vi "APVSG20 module.vi"(10 "Supramodle mailbox":T3) -> ()   [LabVIEW 2024, in "THz source modeule.lvlib"]
doc: "This is a 2024 gen. module for control of AnaPico vector signal generator. \n\nObsolate notes:\nKey typedefs: THz_Message for module, THz_Comands enum (Ignore, Initialize, Update, Set parameters, Disconnect, End), THz_Sweeep parameters\n\nComands and responses:\nInitialize: VDI config constants {Master{lower limit, upper limit, name, handle, description}, Follower{ lower limit, upper limit, name, handle, description } } (cluster of two clusters {numeric, numeric, string, numeric, string}) / handle log (string)\nUpdate: - / M_ID F_ID (string)\nSet parameters: Sweep parameters {Start, End, Sweep up time, Sweep down time, Intermediate, Reset trigger} (cluster{numeric, numeric, numeric, numeric, numeric, boolean}) / Sweep parameters (same cluster)\nDisconnect: - / master and follower name (string)\nEnd: - / Master and Follower handle (string)"
uses:
  THz source modeule.lvlib
  Messenger service/Data types/Module name.ctl
  <vilib>/ErrorRing/Error Ring.xnode
  ctl/APVSG module action.ctl
  <userlib>/MatS Libs/MatS Libs.lvlib
  <userlib>/MatS Libs/MatS Mailman/TypeDefs/General message.ctl
  Magnet module/ctl/Tmp_M commands.ctl
  Magnet module/Magnet module.lvlib
  <userlib>/MatS Libs/MatS Mailman/TypeDefs/Mailbox ref.ctl
  ctl/THz MW generator constants.ctl
  ctl/Module status.ctl
  ctl/THz commands enum.ctl
  <instrlib>/APVSG/APVSG20.lvlib
panel:
  out "Instrument status":T1={"Lower limit [GHz]"=8.0, "Upper limit [GHz]"=20.0, "Device name"="VDIYT7", "Connection"="", "Description"="VDI Tracking", "Connected"=FALSE, "Last settings"="", "Operation mode"=enum."Disabled", "Enable ch 1"=FALSE, "Enable ch 2"=FALSE}
  out "Modul status":T2={"Supramodule"=refnum, "This module"=refnum, "Submodule"=refnum, "Module name"="", "Is standalone"=FALSE, "Timer [ms]"=0, "Reset timer"=TRUE, "Last change"=timestamp(0 s since 1904-01-01), "Logs"=[], "Ended"=FALSE} {"Last change" format="%<%H:%M:%S\n%Y/%m/%d>T"}
  in  "This module mailbox":refnum<queue>
  in  "APVSG tab":enum32{"Status", "CW", "Sweep", "Arbitrary"}(tab)
  in  "Exit APVSG btn":bool
  in  "Connect btn":bool
  in  "Enable ch 2":bool
  in  "Enable ch 1":bool
  in  "VISA resource name":refnum<visa-resource-name>
  out "Is connected":bool
  in  "CW settings":T4(array[cluster])
  in  "Sweep table":T5(array[cluster])
  in  "Waveform files":path[](array[path])
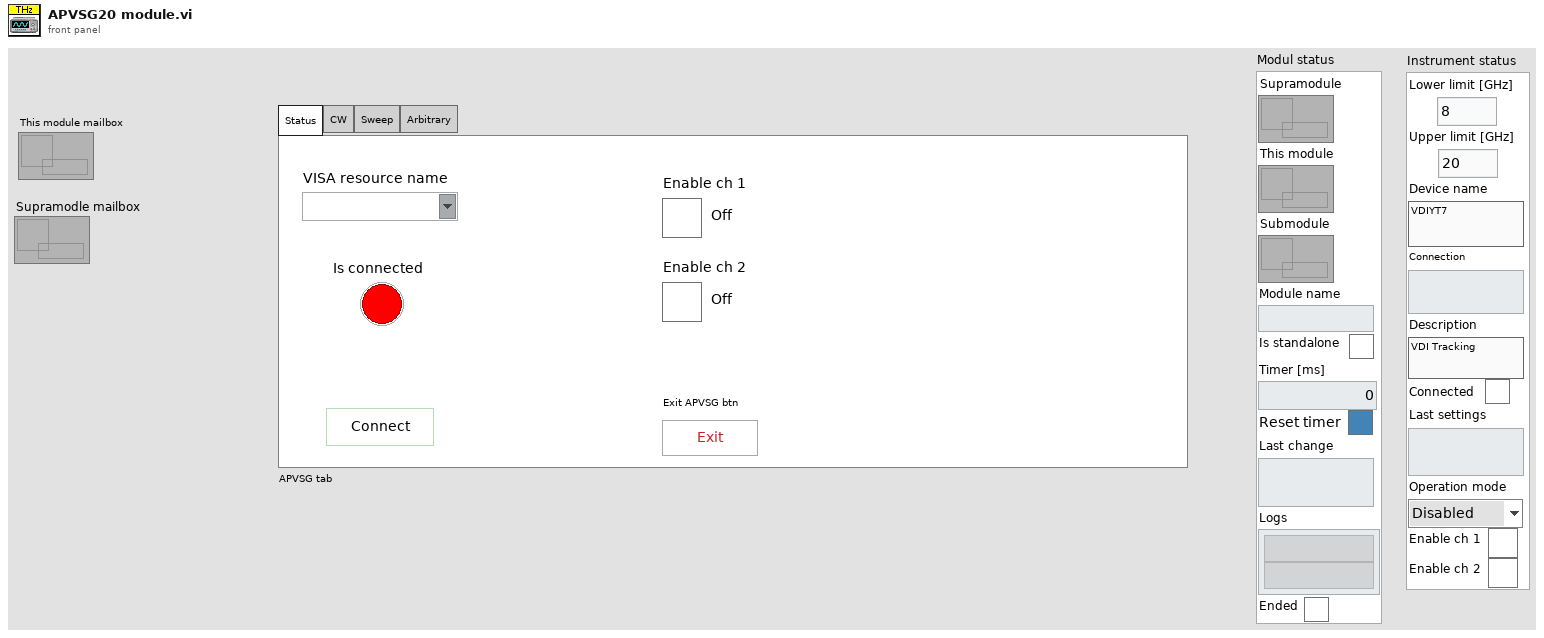
[diagram p1: front panel]
types:
  T1 = typedef "THz source modeule.lvlib/THz MW generator constants.ctl" = cluster{"Lower limit [GHz]":dbl, "Upper limit [GHz]":dbl, "Device name":string, "Connection":string, "Description":string, "Connected":bool, "Last settings":string, "Operation mode":enum16{"Disabled", "CW", "Arbitrary", "Sweep"}, "Enable ch 1":bool, "Enable ch 2":bool}
  T2 = typedef "THz source modeule.lvlib/Module status.ctl" = cluster{"Supramodule":T3, "This module":T3, "Submodule":T3, "Module name":string, "Is standalone":bool, "Timer [ms]":i32, "Reset timer":bool, "Last change":timestamp, "Logs":string[], "Ended":bool}
  T3 = typedef "MatS Libs.lvlib/Mailbox ref.ctl" = refnum<queue>
  T4 = cluster{"Frequency (GHz)":dbl, "Amplitude (dBm)":dbl}[]
  T5 = cluster{"Frequency (GHz)":dbl, "Amplitude (dBm)":dbl, "Time (ns)":dbl}[][]
  T6 = typedef "Module name.ctl" = enum16{"Emty", "Magnet", "VTI", "Excitation", "Servo", "Acquisition", "Rotator", "Digitizer", "SMU2450", "Carousel", "Multimeter", "Tmp monitor", "Power monitor"}
  T7 = cluster{"Supramodule":T3, "This module":T3, "Module name":string, "Standalone?":bool, "Stopped?":bool, "Instr reference":string, "Connected?":bool, "Last update":timestamp, "Logs":string[], "Update period ms":u32}
  T8 = enum16{"Initialize", "Wait for event", "Check message", "Check changes", "End"}
  T9 = typedef "THz source modeule.lvlib/APVSG module action.ctl" = enum16{"Initialize", "Check cmd", "Wait for event", "Connect", "Disconnect", "Query instr", "Set CW", "Set sweep", "Set waveform", "Enable output", "Disable output", "Exit"}
  T10 = enum32{"Bad", "Idle", "Run top level", "Running"}
  T11 = typedef "Magnet module.lvlib/Tmp_M commands.ctl" = enum16{"Ignore", "Log", "Connect", "Set timeout", "Update", "Disconnect", "End"}
  T12 = typedef "MatS Libs.lvlib/General message.ctl" = cluster{"Sender":string, "Recipient":string, "Topic":variant, "Content":variant, "Time Stamp":timestamp}
  T13 = enum16{"Ignore", "Log", "Connect", "Set timeout", "Update", "Disconnect", "End"}
  T14 = enum16{"Ignore", "Log", "Connect", "Set timeout", "Update", "Disconnect", "End"}[]
  T15 = typedef "THz source modeule.lvlib/THz commands enum.ctl" = enum16{"Ignore", "Connect", "Update", "Set parameters", "Disconnect", "End"}
  T16 = enum8{"Enabled", "Disabled", "Disabled and Grayed Out"}
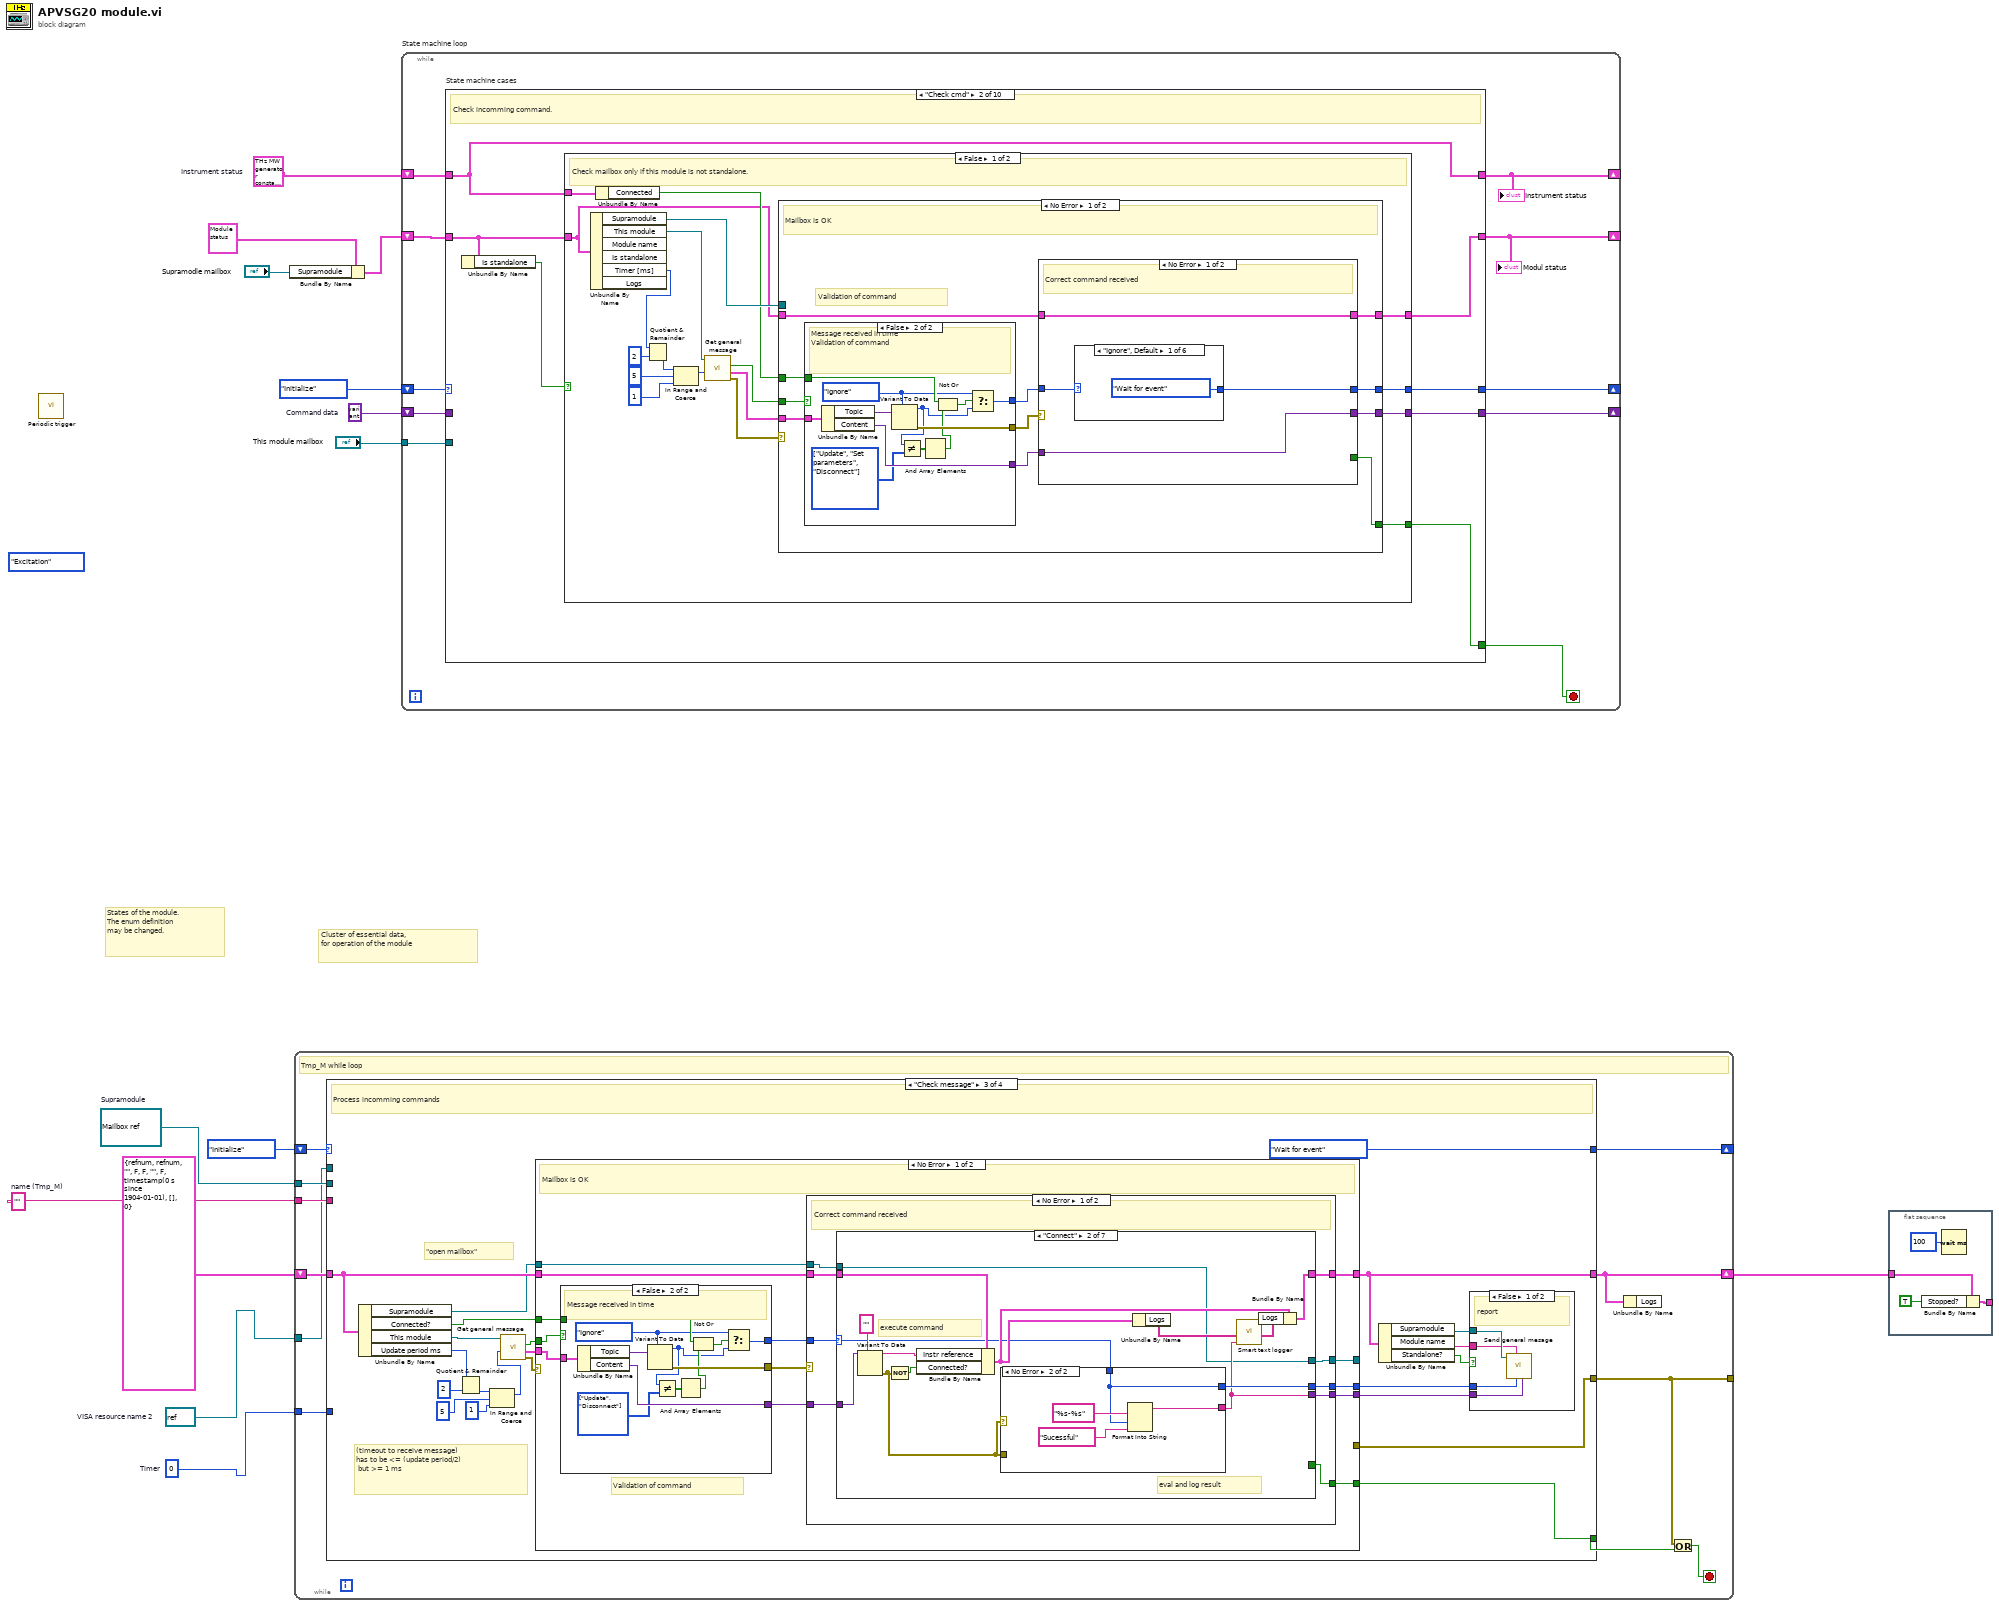
[diagram p0: block diagram]
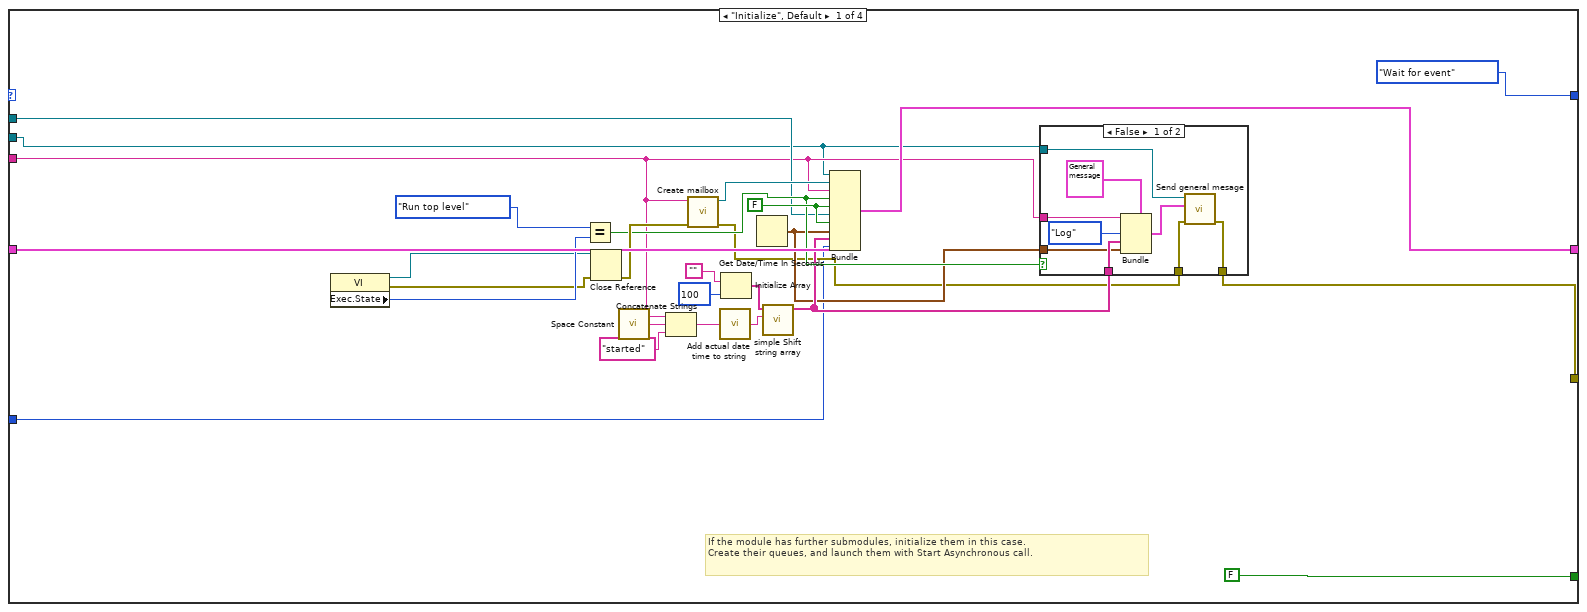
[diagram p2: hidden frame]
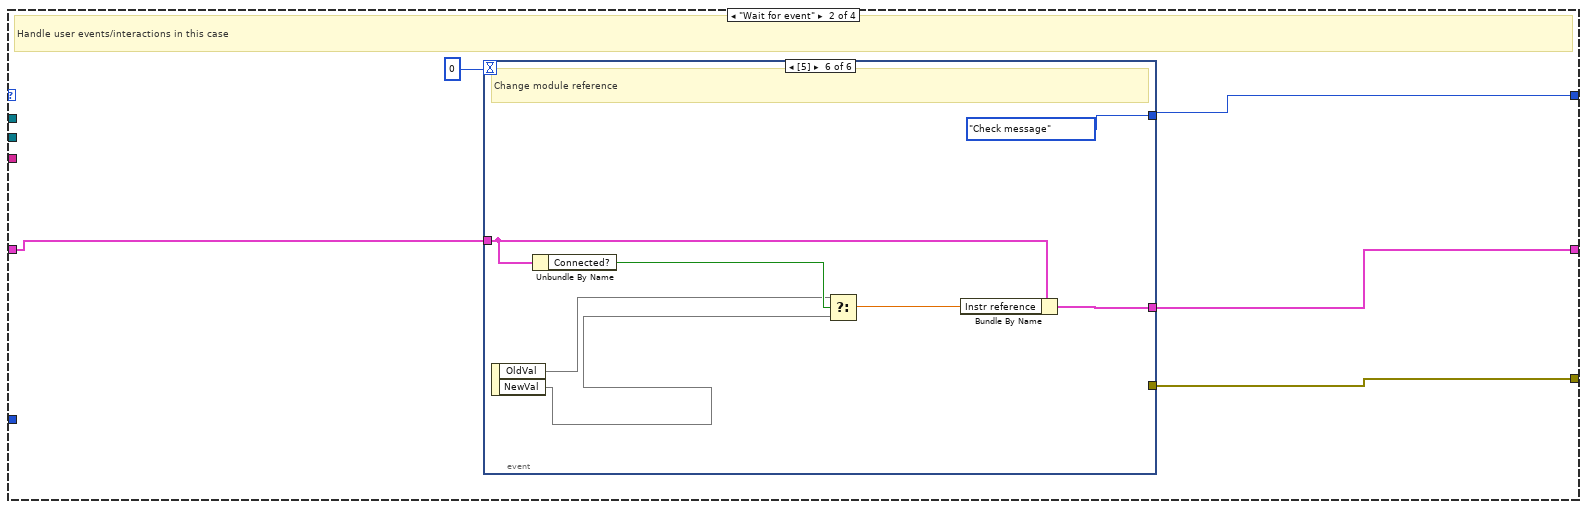
[diagram p4: hidden frame]
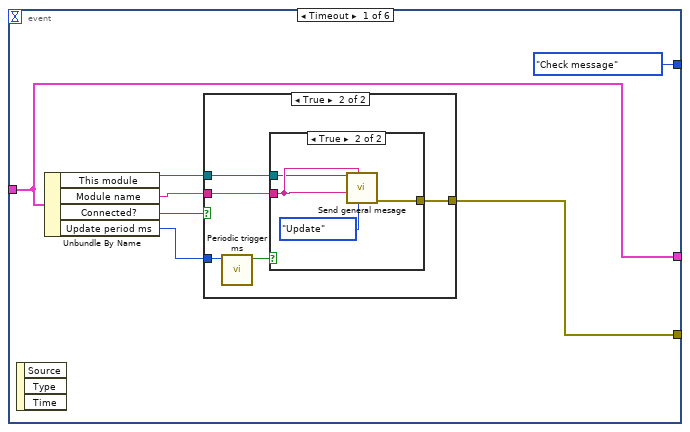
[diagram p5: hidden frame]
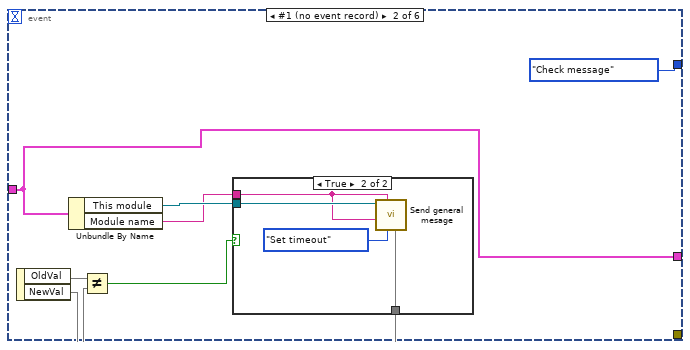
[diagram p8: hidden frame]
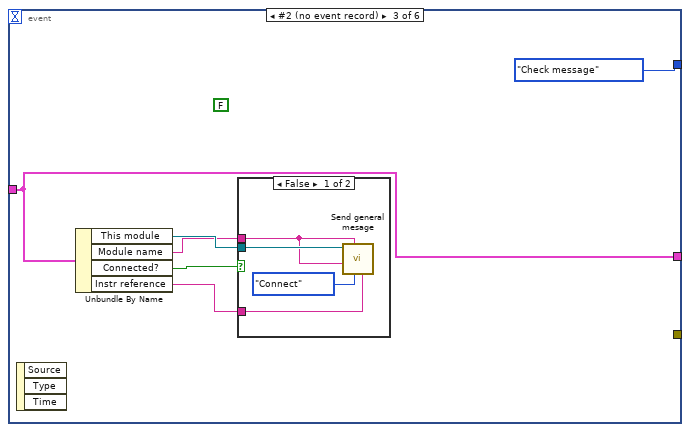
[diagram p10: hidden frame]
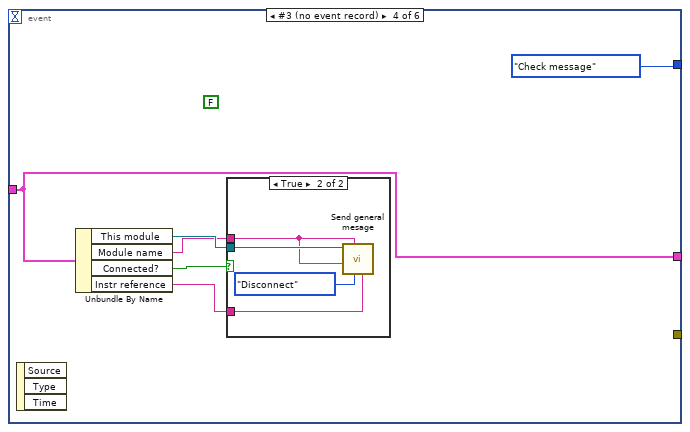
[diagram p12: hidden frame]
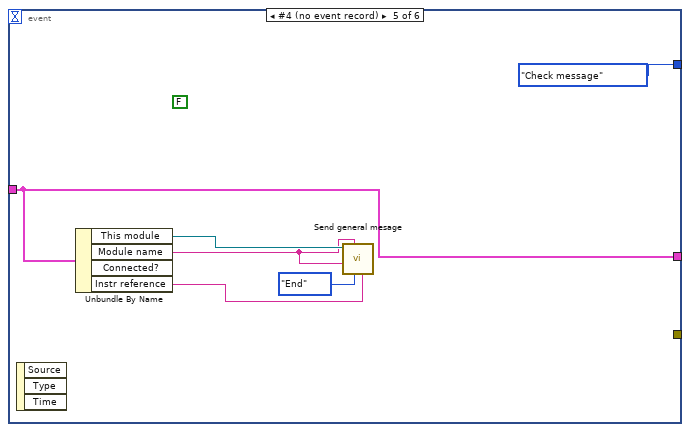
[diagram p14: hidden frame]
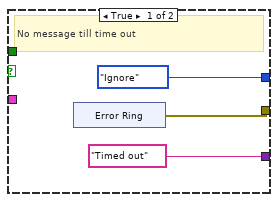
[diagram p16: hidden frame]
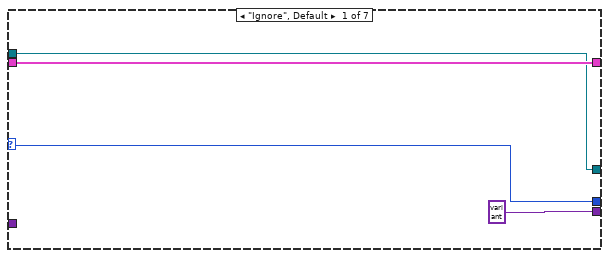
[diagram p17: hidden frame]
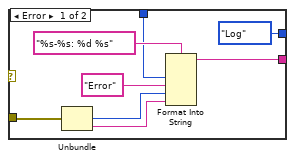
[diagram p18: hidden frame]
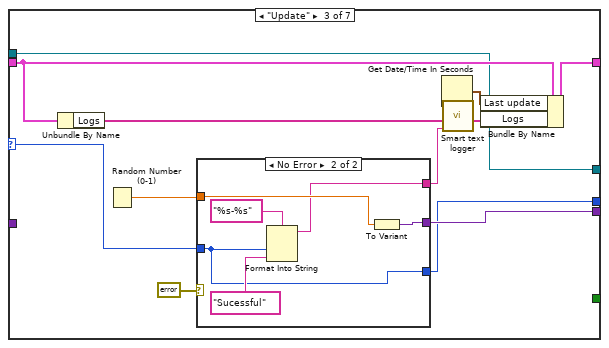
[diagram p19: hidden frame]
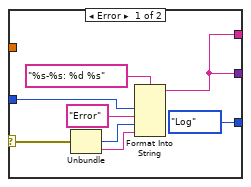
[diagram p20: hidden frame]
diagram:
  (unwired) Module_name."Excitation" ("Module")
  w3 = T1 {"Lower limit [GHz]"=8.0, "Upper limit [GHz]"=20.0, "Device name"="VDIYT7", "Connection"="", "Description"="VDI Tracking", "Connected"=FALSE, "Last settings"="", "Operation mode"=enum."Disabled", "Enable ch 1"=FALSE, "Enable ch 2"=FALSE}  # Instrument status
  w4 = variant  # Command data
  w11 = 0  # Timer
  w10 = refnum<visa-resource-name> refnum  # VISA resource name 2
  w9 = ""  # name (Tmp_M)
  w8 = T3 refnum  # Supramodule
  # "States of the module.\nThe enum definition\nmay be changed."
  # "Cluster of essential data,\nfor operation of the module"
  n1 = call <userlib>:"Periodic trigger.vi"() -> ()  [unwired: 3 in, 1 out]
  n2 = Bundle By Name(cluster=T2 {"Supramodule"=refnum, "This module"=refnum, "Submodule"=refnum, "Module name"="Signal generator", "Is standalone"=FALSE, "Timer [ms]"=5000, "Reset timer"=FALSE, "Last change"=timestamp(0 s since 1904-01-01), "Logs"=[], "Ended"=FALSE}, "Supramodule"="Supramodle mailbox") -> (w2:T2)
  n3 = while {
    tunnel: [w19] -> _
    shift-right: [w23] -> _
    shift-left: T8."Initialize" -> [w24]
    shift-right: [w20] -> w6
    shift-left: T7 {"Supramodule"=refnum, "This module"=refnum, "Module name"="", "Standalone?"=FALSE, "Stopped?"=FALSE, "Instr reference"="", "Connected?"=FALSE, "Last update"=timestamp(0 s since 1904-01-01), "Logs"=[], "Update period ms"=0} ("Module status") -> [w22]
    tunnel: w9 -> [w18]
    tunnel: w8 -> [w17]
    tunnel: w11 -> [w16]
    tunnel: w10 -> [w15]
    stop <- w21 stop-if-true
    # "Tmp_M while loop"
    n4 = case shown="\"Check message\"" w24 {
      tunnel: [FALSE _ w149 _] -> w25
      tunnel: [w30 w65 w130 _] -> w19
      tunnel: [T8."Wait for event" w67 T8."Wait for event" T8."End"] -> w23
      tunnel: w22 -> [w50 w63 w147 w374]
      tunnel: [w48 w64 w133 w374] -> w20
      tunnel: w15 -> [w29 _ _ _]
      tunnel: w18 -> [w28 _ _ _]
      tunnel: w17 -> [w27 _ _ _]
      tunnel: w16 -> [w26 _ _ _]
      frame "Initialize", Default {
        w47 = FALSE ("Connected?")
        # "If the module has further submodules, initialize them in this case.\nCreate their queues, and launch them with Start Asynchronous call."
        n5 = property class="VI"() -> (reference out=w38:refnum<vi>, error out=w37:errorcluster, "Exec.State"=w40:T10)  [unwired: 2 in]
        n6 = Equal?(x=T10."Run top level" ("y"), y=w40) -> (x = y?=w34:bool)
        n7 = Close Reference(reference=w38, error in (no error)=w37) -> (error out=w36:errorcluster)
        n8 = call <vilib>:"Space Constant.vi"() -> ("String"=w46:string)
        n9 = Concatenate Strings(w28, w46, "started") -> (w45:string)
        n10 = call <userlib>:"Create mailbox.vi"("error in (no error)"=w36, "name (unnamed)"=w28) -> ("error out"=w31:errorcluster, "Mailbox ref"=w49:T3)  [unwired: 3 in, 1 out]
        n11 = call <userlib>:"Add actual date time to string.vi"("String in"=w45) -> ("String out"=w35:string)  [unwired: 4 in]
        n12 = Initialize Array("", 100 ("dimension size")) -> (w41:string[])
        n13 = Get Date/Time In Seconds() -> (seconds since 1Jan1904=w32:timestamp)
        n14 = call <userlib>:"simple Shift string array.vi"("Element in"=w35, "Array in"=w41) -> ("Array out"=w33:string[])  [unwired: 8 in, 1 out]
        n15 = Bundle(cluster=w50, "Supramodule"=w27, "This module"=w49, "Module name"=w28, "Standalone?"=w34, "Stopped?"=w47, "Instr reference"=w29, "Connected?"=w47, "Last update"=w32, "Logs"=w33, "Update period ms"=w26) -> (w48:T7)
        n16 = case shown="False" w34 {
          tunnel: w27 -> [w61 _]
          tunnel: w33 -> [w59 _]
          tunnel: w32 -> [w58 _]
          tunnel: w28 -> [w56 _]
          tunnel: w31 -> [w55 w62]
          tunnel: [w54 w62] -> w30
          frame False {
            n17 = Bundle(cluster=T12 {"Sender"="", "Recipient"="", "Topic"=variant(string ""), "Content"=variant, "Time Stamp"=timestamp(0 s since 1904-01-01)} ("Message"), "Sender"=w56, "Topic"=Tmp_M_commands."Log" ("Command"), "Content"=w59, "Time Stamp"=w58) -> (w57:T12)  [unwired: 1 in]
            n18 = call <userlib>:"Send general mesage.vi"("error in (no error)"=w55, "Message"=w57, "Mailbox ref in"=w61) -> ("error out"=w54:errorcluster)  [unwired: 6 in, 2 out]
          }
          frame True {
          }
        }
      }
      frame "Wait for event" {
        # "Handle user events/interactions in this case"
        n19 = event shown="[5]" {
          selector: _ -> [_ _ _ _ _ _]
          dyn-events: _ -> [_ _ _ _ _ _]
          timeout: 0 -> [_ _ _ _ _ _]
          tunnel: [T8."Check message" T8."Check message" T8."Check message" T8."Check message" T8."Check message" T8."Check message"] -> w67
          tunnel: [w73 _ _ _ _ _] -> w65
          tunnel: w63 -> [w71 w90 w100 w110 w120 w127]
          tunnel: [w71 w90 w100 w110 w120 w126] -> w64
          event Timeout {
            n20 = event-data() -> ()  [unwired: 1 in, 3 out]
            n21 = Unbundle By Name(w71) -> ("This module"=w69:T3, "Module name"=w70:string, "Connected?"=w72:bool, "Update period ms"=w68:u32)
            n22 = case shown="True" w72 {
              tunnel: w68 -> [_ w79]
              tunnel: [_ w78] -> w73
              tunnel: w70 -> [_ w76]
              tunnel: w69 -> [_ w75]
              frame False {
              }
              frame True {
                n23 = call <userlib>:"Periodic trigger ms.vi"("Period ms"=w79) -> ("Trigger"=w77:bool)  [unwired: 6 in]
                n24 = case shown="True" w77 {
                  tunnel: [_ w83] -> w78
                  tunnel: w76 -> [_ w82]
                  tunnel: w75 -> [_ w81]
                  frame False {
                  }
                  frame True {
                    n25 = call <userlib>:"Send general mesage.vi"("Topic"=Tmp_M_commands."Update" ("Command"), "Sender"=w82, "Recipient"=w82, "Mailbox ref in"=w81) -> ("error out"=w83:errorcluster)  [unwired: 5 in, 2 out]
                  }
                }
              }
            }
          }
          event #1 (no event record) {
            n26 = event-data() -> ("OldVal"=w87, "NewVal"=w84)  [unwired: 1 in]
            n27 = Unbundle By Name(w90) -> ("This module"=w89:T3, "Module name"=w88:string)
            n28 = Not Equal?(x=w87, y=w84) -> (x != y?=w86:bool)
            n29 = case shown="True" w86 {
              tunnel: w89 -> [_ w94]
              tunnel: w88 -> [_ w93]
              tunnel: w84 -> [_ w91]
              frame False {
              }
              frame True {
                n30 = call <userlib>:"Send general mesage.vi"("Content"=w91, "Topic"=T13."Set timeout" ("Command"), "Sender"=w93, "Recipient"=w93, "Mailbox ref in"=w94) -> ()  [unwired: 4 in, 3 out]
              }
            }
          }
          event #2 (no event record) {
            (unwired) FALSE ("Connect btn 3")
            n31 = event-data() -> ()  [unwired: 1 in, 3 out]
            n32 = Unbundle By Name(w100) -> ("This module"=w98:T3, "Module name"=w97:string, "Connected?"=w99:bool, "Instr reference"=w96:string)
            n33 = case shown="False" w99 {
              tunnel: w98 -> [w104 _]
              tunnel: w97 -> [w103 _]
              tunnel: w96 -> [w101 _]
              frame False {
                n34 = call <userlib>:"Send general mesage.vi"("Content"=w101, "Topic"=Tmp_M_commands."Connect" ("Command"), "Sender"=w103, "Recipient"=w103, "Mailbox ref in"=w104) -> ()  [unwired: 4 in, 3 out]
              }
              frame True {
              }
            }
          }
          event #3 (no event record) {
            (unwired) FALSE ("Disconnect btn")
            n35 = event-data() -> ()  [unwired: 1 in, 3 out]
            n36 = Unbundle By Name(w110) -> ("This module"=w108:T3, "Module name"=w107:string, "Connected?"=w109:bool, "Instr reference"=w106:string)
            n37 = case shown="True" w109 {
              tunnel: w108 -> [_ w114]
              tunnel: w107 -> [_ w113]
              tunnel: w106 -> [_ w111]
              frame False {
              }
              frame True {
                n38 = call <userlib>:"Send general mesage.vi"("Content"=w111, "Topic"=Tmp_M_commands."Disconnect" ("Command"), "Sender"=w113, "Recipient"=w113, "Mailbox ref in"=w114) -> ()  [unwired: 4 in, 3 out]
              }
            }
          }
          event #4 (no event record) {
            (unwired) FALSE ("Stop btn")
            n39 = event-data() -> ()  [unwired: 1 in, 3 out]
            n40 = Unbundle By Name(w120) -> ("This module"=w119:T3, "Module name"=w118:string, "Instr reference"=w117:string)  [unwired: 1 out]
            n41 = call <userlib>:"Send general mesage.vi"("Content"=w117, "Topic"=Tmp_M_commands."End" ("Command"), "Sender"=w118, "Recipient"=w118, "Mailbox ref in"=w119) -> ()  [unwired: 4 in, 3 out]
          }
          event #5 (no event record) {
            # "Change module reference"
            n42 = event-data() -> ("OldVal"=w124, "NewVal"=w121)  [unwired: 1 in]
            n43 = Unbundle By Name(w127) -> ("Connected?"=w125:bool)
            n44 = Select(t=w124, s=w125, f=w121) -> (s? t:f=w122:dbl)
            n45 = Bundle By Name(cluster=w127, "Instr reference"=w122) -> (w126:T7)
          }
        }
      }
      frame "Check message" {
        # "\"open mailbox\""
        # "(timeout to receive message)\nhas to be <= (update period/2)\n but >= 1 ms"
        # "Process incomming commands"
        n46 = Unbundle By Name(w147) -> ("Supramodule"=w129:T3, "Connected?"=w136:bool, "This module"=w140:T3, "Update period ms"=w145:u32)
        n47 = Quotient & Remainder(x=w145, y=u32 2) -> (floor(x/y)=w143:u32)  [unwired: 1 out]
        n48 = In Range and Coerce(upper limit=w143, x=u32 5, lower limit=u32 1) -> (coerced(x)=w139:u32)  [unwired: 1 out]
        n49 = call <userlib>:"Get general message.vi"("timeout ms (1000)"=w139, "Mailbox ref in"=w140) -> ("error out"=w138:errorcluster, "Message"=w141:T12, "timed out?"=w137:bool)  [unwired: 4 in, 3 out]
        n50 = case shown="No Error" w138 {
          selector: w138 -> [_ w366]
          tunnel: [w166 TRUE] -> w149
          tunnel: [w165 w372] -> w133
          tunnel: w147 -> [w164 w372]
          tunnel: w141 -> [w163 _]
          tunnel: w137 -> [w160 _]
          tunnel: w136 -> [w158 _]
          tunnel: [w157 Tmp_M_commands."End" ("Cmd out")] -> w132
          tunnel: [w156 w367] -> w131
          tunnel: [_ w366] -> w130
          tunnel: [w155 w365] -> _
          tunnel: w129 -> [w154 w365]
          frame No Error {
            # "Validation of command"
            # "Mailbox is OK"
            n51 = case shown="False" w160 {
              tunnel: w163 -> [_ w182]
              tunnel: [w168 w180] -> w162
              tunnel: [T13."Ignore" ("Command") w178] -> w161
              tunnel: ["Timed out" w179] -> w159
              tunnel: w158 -> [_ w176]
              frame True {
                # "No message till time out"
                n52 = xnode "Error Ring"() -> ("error out"=w168:errorcluster)
              }
              frame False {
                w175 = T14 [enum."Update", enum."Disconnect"] items=["Ignore", "Log", "Connect", "Set timeout", "Update", "Disconnect", "End"] ("Command")
                w172 = T13."Ignore" ("Command")
                # "Message received in time"
                n53 = Unbundle By Name(w182) -> ("Topic"=w181:variant, "Content"=w179:variant)
                n54 = Variant To Data(type=w172, Variant=w181) -> (data=w171:T13, error out=w180:errorcluster)  [unwired: 1 in]
                n55 = Not Equal?(x=w171, y=w175) -> (x != y?=w174:bool[])
                n56 = And Array Elements(Boolean array=w174) -> (logical AND=w173:bool)
                n57 = Not Or(1:w173, 2:w176) -> (0:w177:bool)
                n58 = Select(t=w172, s=w177, f=w171) -> (s? t:f=w178:T13)
              }
            }
            n59 = case shown="No Error" w162 {
              selector: w162 -> [_ w363]
              tunnel: [w187 FALSE] -> w166
              tunnel: [w191 w362] -> w165
              tunnel: w164 -> [w190 w359]
              tunnel: w161 -> [w188 _]
              tunnel: w159 -> [w189 _]
              tunnel: [w186 Tmp_M_commands."Log" ("Command")] -> w157
              tunnel: [w185 w354] -> w156
              tunnel: [w184 w353] -> w155
              tunnel: w154 -> [w183 w353]
              frame No Error {
                # "Correct command received"
                n60 = case shown="\"Connect\"" w188 {
                  selector: w188 -> [w193 w200 w225 w252 w278 w302 w328]
                  tunnel: [_ _ _ _ w275 _ FALSE] -> w187
                  tunnel: [w195 w202 w233 w258 w283 w306 w330] -> w191
                  tunnel: w190 -> [w195 w207 w232 w257 w282 w305 w334]
                  tunnel: w189 -> [_ w206 _ _ _ w304 w333]
                  tunnel: [w193 w198 w223 w251 w277 w301 w327] -> w186
                  tunnel: [variant w197 w227 w250 w276 w300 w325] -> w185
                  tunnel: [w192 w196 w222 w248 w272 w297 w324] -> w184
                  tunnel: w183 -> [w192 w196 w222 w248 w272 w297 w324]
                  frame "Ignore", Default {
                  }
                  frame "Connect" {
                    # "eval and log result"
                    # "execute command"
                    n61 = Variant To Data(type="", Variant=w206) -> (data=w208:string, error out=w199:errorcluster)  [unwired: 1 in]
                    n62 = Not(x=w199) -> (.not. x?=w201:bool)
                    n63 = Bundle By Name(cluster=w207, "Instr reference"=w208, "Connected?"=w201) -> (w203:T7)
                    n64 = case shown="No Error" w199 {
                      tunnel: [w213 w219] -> w197
                      tunnel: w199 -> [w212 _]
                      tunnel: w200 -> [w211 w218]
                      tunnel: [T13."Log" ("Command") w218] -> w198
                      frame Error {
                        n65 = Unbundle(w212) -> ("code"=w216:i32, "source"=w215:string)  [unwired: 1 out]
                        n66 = Format Into String(format string="%s-%s: %d %s" ("f"), w211, "Error" ("f"), w216, w215) -> (resulting string=w213:string)  [unwired: 2 in, 1 out]
                      }
                      frame No Error {
                        n67 = Format Into String(format string="%s-%s" ("f"), w218, "Sucessful" ("f")) -> (resulting string=w219:string)  [unwired: 2 in, 1 out]
                      }
                    }
                    n68 = Unbundle By Name(w203) -> ("Logs"=w205:string[])
                    n69 = call <userlib>:"Smart text logger.vi"("Message"=w197, "Logs in"=w205) -> ("Logs out"=w204:string[])  [unwired: 8 in, 1 out]
                    n70 = Bundle By Name(cluster=w203, "Logs"=w204) -> (w202:T7)
                  }
                  frame "Update" {
                    n71 = Unbundle By Name(w232) -> ("Logs"=w229:string[])
                    n72 = Random Number (0-1)() -> (number: 0 to 1=w228:dbl)
                    n73 = case shown="No Error" errorcluster {"status"=FALSE, "code"=0, "source"=""} ("error IO") {
                      selector: errorcluster {"status"=FALSE, "code"=0, "source"=""} ("error IO") -> [w235 _]
                      tunnel: [w234 w242] -> w226
                      tunnel: w225 -> [w237 w245]
                      tunnel: [T13."Log" ("Command") w245] -> w223
                      tunnel: [w234 w244] -> w227
                      tunnel: w228 -> [_ w243]
                      frame Error {
                        n74 = Unbundle(w235) -> ("code"=w240:i32, "source"=w239:string)  [unwired: 1 out]
                        n75 = Format Into String(format string="%s-%s: %d %s" ("f"), w237, "Error" ("f"), w240, w239) -> (resulting string=w234:string)  [unwired: 2 in, 1 out]
                      }
                      frame No Error {
                        n76 = Format Into String(format string="%s-%s" ("f"), w245, "Sucessful" ("f")) -> (resulting string=w242:string)  [unwired: 2 in, 1 out]
                        n77 = To Variant(anything=w243) -> (Variant=w244:variant)
                      }
                    }
                    n78 = Get Date/Time In Seconds() -> (seconds since 1Jan1904=w231:timestamp)
                    n79 = call <userlib>:"Smart text logger.vi"("Message"=w226, "Logs in"=w229) -> ("Logs out"=w230:string[])  [unwired: 8 in, 1 out]
                    n80 = Bundle By Name(cluster=w232, "Last update"=w231, "Logs"=w230) -> (w233:T7)
                  }
                  frame "Disconnect" {
                    n81 = Unbundle By Name(w257) -> ("Logs"=w254:string[])
                    n82 = case shown="Error .." errorcluster {"status"=FALSE, "code"=0, "source"=""} ("error IO") {
                      selector: errorcluster {"status"=FALSE, "code"=0, "source"=""} ("error IO") -> [w260 _]
                      tunnel: w252 -> [w262 w269]
                      tunnel: [T13."Log" ("Command") w269] -> w251
                      tunnel: [w259 w268] -> w250
                      tunnel: [w259 w267] -> w249
                      frame Error {
                        n83 = Unbundle(w260) -> ("code"=w265:i32, "source"=w264:string)  [unwired: 1 out]
                        n84 = Format Into String(format string="%s-%s: %d %s" ("f"), w262, "Error" ("f"), w265, w264) -> (resulting string=w259:string)  [unwired: 2 in, 1 out]
                      }
                      frame No Error {
                        n85 = Format Into String(format string="%s-%s" ("f"), w269, "Sucessful" ("f")) -> (resulting string=w267:string)  [unwired: 2 in, 1 out]
                        n86 = To Variant(anything=w267) -> (Variant=w268:variant)
                      }
                    }
                    n87 = call <userlib>:"Smart text logger.vi"("Message"=w249, "Logs in"=w254) -> ("Logs out"=w255:string[])  [unwired: 8 in, 1 out]
                    n88 = Bundle By Name(cluster=w257, "Connected?"=FALSE, "Logs"=w255) -> (w258:T7)
                  }
                  frame "End" {
                    w274 = errorcluster {"status"=FALSE, "code"=0, "source"=""} ("error IO")
                    n89 = case shown="Error .." w274 {
                      selector: w274 -> [w285 _]
                      tunnel: [w284 w292] -> w273
                      tunnel: w278 -> [w287 w294]
                      tunnel: [T13."Log" ("Command") w294] -> w277
                      tunnel: [w284 w293] -> w276
                      frame Error {
                        n90 = Unbundle(w285) -> ("code"=w290:i32, "source"=w289:string)  [unwired: 1 out]
                        n91 = Format Into String(format string="%s-%s: %d %s" ("f"), w287, "Error" ("f"), w290, w289) -> (resulting string=w284:string)  [unwired: 2 in, 1 out]
                      }
                      frame No Error {
                        n92 = Format Into String(format string="%s-%s" ("f"), w294, "Sucessful" ("f")) -> (resulting string=w292:string)  [unwired: 2 in, 1 out]
                        n93 = To Variant(anything=w292) -> (Variant=w293:variant)
                      }
                    }
                    n94 = Unbundle By Name(w282) -> ("Logs"=w279:string[])
                    n95 = call <userlib>:"Smart text logger.vi"("Message"=w273, "Logs in"=w279) -> ("Logs out"=w280:string[])  [unwired: 8 in, 1 out]
                    n96 = Bundle By Name(cluster=w282, "Connected?"=FALSE, "Logs"=w280) -> (w283:T7)
                    n97 = Not(x=w274) -> (.not. x?=w275:bool)
                  }
                  frame "Log" {
                    n98 = Variant To Data(type="", Variant=w304) -> (data=w299:string, error out=w303:errorcluster)  [unwired: 1 in]
                    n99 = case shown="Error .." w303 {
                      selector: w303 -> [w311 _]
                      tunnel: [w310 w318] -> w298
                      tunnel: w302 -> [w313 w321]
                      tunnel: [T13."Log" ("Command") w321] -> w301
                      tunnel: [w310 w320] -> w300
                      tunnel: w299 -> [_ w318]
                      frame Error {
                        n100 = Unbundle(w311) -> ("code"=w316:i32, "source"=w315:string)  [unwired: 1 out]
                        n101 = Format Into String(format string="%s-%s: %d %s" ("f"), w313, "Error" ("f"), w316, w315) -> (resulting string=w310:string)  [unwired: 2 in, 1 out]
                      }
                      frame No Error {
                        n102 = Format Into String(format string="%s-%s" ("f"), w321, "Sucessful" ("f")) -> (resulting string=w319:string)  [unwired: 2 in, 1 out]
                        n103 = To Variant(anything=w319) -> (Variant=w320:variant)
                      }
                    }
                    n104 = Unbundle By Name(w305) -> ("Logs"=w307:string[])
                    n105 = call <userlib>:"Smart text logger.vi"("Message"=w298, "Logs in"=w307) -> ("Logs out"=w308:string[])  [unwired: 8 in, 1 out]
                    n106 = Bundle By Name(cluster=w305, "Logs"=w308) -> (w306:T7)
                  }
                  frame "Set timeout" {
                    n107 = Variant To Data(type=0 ("timeout ms"), Variant=w333) -> (data=w336:i32, error out=w329:errorcluster)  [unwired: 1 in]
                    n108 = Bundle By Name(cluster=w334, "Update period ms"=w336) -> (w332:T7)
                    n109 = case shown="Error .." w329 {
                      selector: w329 -> [w340 _]
                      tunnel: [w339 w350] -> w326
                      tunnel: w328 -> [w342 w349]
                      tunnel: [T13."Log" ("Command") w349] -> w327
                      tunnel: [w339 w348] -> w325
                      tunnel: w336 -> [_ w347]
                      frame Error {
                        n110 = Unbundle(w340) -> ("code"=w345:i32, "source"=w344:string)  [unwired: 1 out]
                        n111 = Format Into String(format string="%s-%s: %d %s" ("f"), w342, "Error" ("f"), w345, w344) -> (resulting string=w339:string)  [unwired: 2 in, 1 out]
                      }
                      frame No Error {
                        n112 = To Variant(anything=w347) -> (Variant=w348:variant)
                        n113 = Format Into String(format string="%s-%s: %d ms" ("f"), w349, "Sucessful" ("f"), w347) -> (resulting string=w350:string)  [unwired: 2 in, 1 out]
                      }
                    }
                    n114 = Unbundle By Name(w332) -> ("Logs"=w335:string[])
                    n115 = call <userlib>:"Smart text logger.vi"("Message"=w326, "Logs in"=w335) -> ("Logs out"=w331:string[])  [unwired: 8 in, 1 out]
                    n116 = Bundle By Name(cluster=w332, "Logs"=w331) -> (w330:T7)
                  }
                }
              }
              frame Error {
                # "Unknown command received"
                n117 = Unbundle(w363) -> ("code"=w356:i32, "source"=w357:string)  [unwired: 1 out]
                n118 = Format Into String(format string="Unknown command Error: %d %s", w356, w357) -> (resulting string=w354:string)  [unwired: 2 in, 1 out]
                n119 = Unbundle By Name(w359) -> ("Logs"=w360:string[])
                n120 = call <userlib>:"Smart text logger.vi"("Message"=w354, "Logs in"=w360) -> ("Logs out"=w361:string[])  [unwired: 8 in, 1 out]
                n121 = Bundle By Name(cluster=w359, "Logs"=w361) -> (w362:T7)
              }
            }
          }
          frame Error {
            # "Queue Error"
            n122 = Unbundle(w366) -> ("code"=w370:i32, "source"=w369:string)  [unwired: 1 out]
            n123 = Format Into String(format string="Queue Error: %d %s" ("f"), w370, w369) -> (resulting string=w367:string)  [unwired: 2 in, 1 out]
          }
        }
        n124 = Unbundle By Name(w133) -> ("Supramodule"=w135:T3, "Module name"=w134:string, "Standalone?"=w128:bool)
        n125 = case shown="False" w128 {
          tunnel: w135 -> [w153 _]
          tunnel: w134 -> [w152 _]
          tunnel: w132 -> [w151 _]
          tunnel: w131 -> [w150 _]
          frame False {
            # "report"
            n126 = call <userlib>:"Send general mesage.vi"("Content"=w150, "Topic"=w151, "Sender"=w152, "Mailbox ref in"=w153) -> ()  [unwired: 5 in, 3 out]
          }
          frame True {
          }
        }
      }
      frame "End" {
      }
    }
    n127 = Unbundle By Name(w20) -> ()  [unwired: 1 out]
    n128 = Or(x=w19, y=w25) -> (x .or. y?=w21:bool)
  }
  n129 = while "State machine loop" {
    shift-right: [w384] -> _
    shift-left: APVSG_module_action."Initialize" -> [w385]
    shift-right: [w382] -> _
    shift-left: w2 -> [w383]
    tunnel: "This module mailbox" -> [w381]
    shift-right: [w380] -> _
    shift-left: w4 -> [w379]
    shift-right: [w377] -> _
    shift-left: w3 -> [w378]
    stop <- w376 stop-if-true
    n130 = case "State machine cases" shown="\"Check cmd\"" w385 {
      selector: w385 -> [_ _ _ w589 w614 w632 w653 _ _ _]
      tunnel: [APVSG_module_action."Check cmd" w420 w521 APVSG_module_action."Wait for event" APVSG_module_action."Check cmd" _ APVSG_module_action."Wait for event" _ _ _] -> w384
      tunnel: w383 -> [w394 w418 w510 w586 w611 w635 w668 w701 w703 w707]
      tunnel: [w393 w422 w514 w585 w610 w646 w666 w701 w703 w708] -> w382
      tunnel: w381 -> [w386 _ _ _ _ _ _ _ _ _]
      tunnel: [variant ("Data") w421 w506 variant ("Data") variant ("Data") _ variant _ _ _] -> w380
      tunnel: w379 -> [_ _ _ w593 _ _ w671 _ _ w712]
      tunnel: w378 -> [w395 w423 w505 w573 w604 w636 w667 w702 w704 w711]
      tunnel: [w395 w423 w505 w582 w603 w631 w665 w702 w704 w709] -> w377
      tunnel: [_ w419 _ _ _ _ _ _ _ _] -> w376
      frame "Initialize", Default {
        (unwired) APVSG_module_action."Initialize"
        # "In this state GUI, and internal status of module should be initialized."
        n131 = Get Queue Status(queue=w386) -> ()  [unwired: 2 in, 8 out]
        n132 = Select() -> ()  [unwired: 3 in, 1 out]
        n133 = property class="VI"() -> (reference out=w405:refnum<vi>, error out=w406:errorcluster, "Exec.State"=w403:T10)  [unwired: 2 in]
        n134 = Unbundle By Name(w394) -> ("Supramodule"=w389:T3, "Module name"=w388:string)
        n135 = Equal?(x=T10."Run top level" ("y"), y=w403) -> (x = y?=w392:bool)
        n136 = Close Reference(reference=w405, error in (no error)=w406) -> (error out=w407:errorcluster)
        n137 = call <vilib>:"Space Constant.vi"() -> ("String"=w397:string)
        n138 = call <userlib>:"Create mailbox.vi"("error in (no error)"=w407, "name (unnamed)"=w388) -> ("Mailbox ref"=w396:T3)  [unwired: 3 in, 2 out]
        n139 = Concatenate Strings(w388, w397, "started") -> (w398:string)
        n140 = call <userlib>:"Add actual date time to string.vi"("String in"=w398) -> ("String out"=w391:string)  [unwired: 4 in]
        n141 = Initialize Array("", 100 ("dimension size")) -> (w402:string[])
        n142 = Get Date/Time In Seconds() -> (seconds since 1Jan1904=w390:timestamp)
        n143 = call <userlib>:"simple Shift string array.vi"("Element in"=w391, "Array in"=w402) -> ("Array out"=w408:string[])  [unwired: 8 in, 1 out]
        n144 = Bundle By Name(cluster=w394, "This module"=w396, "Is standalone"=w392, "Last change"=w390, "Logs"=w408) -> (w393:T2)
        n145 = case shown="False" w392 {
          tunnel: w389 -> [w416 _]
          tunnel: w391 -> [w412 _]
          tunnel: w390 -> [w411 _]
          tunnel: w388 -> [w410 _]
          frame False {
            n146 = Bundle(cluster=T12 {"Sender"="", "Recipient"="", "Topic"=variant(string ""), "Content"=variant, "Time Stamp"=timestamp(0 s since 1904-01-01)} ("Message"), "Sender"=w410, "Topic"=Tmp_M_commands."Log" ("Command"), "Content"=w412, "Time Stamp"=w411) -> (w414:T12)  [unwired: 1 in]
            n147 = call <userlib>:"Send general mesage.vi"("Message"=w414, "Mailbox ref in"=w416) -> ()  [unwired: 7 in, 3 out]
          }
          frame True {
          }
        }
      }
      frame "Check cmd" {
        # "Check incomming command."
        n148 = Unbundle By Name(w418) -> ("Is standalone"=w417:bool)
        n149 = case shown="False" w417 {
          tunnel: w423 -> [w438 _]
          tunnel: [w428 w504] -> w422
          tunnel: w418 -> [w427 w504]
          tunnel: [w426 variant ("Content")] -> w421
          tunnel: [w425 APVSG_module_action."Wait for event"] -> w420
          tunnel: [w424 _] -> w419
          frame False {
            # "Check mailbox only if this module is not standalone."
            n150 = Unbundle By Name(w427) -> ("Supramodule"=w433:T3, "This module"=w435:T3, "Timer [ms]"=w441:i32)  [unwired: 3 out]
            n151 = Unbundle By Name(w438) -> ("Connected"=w429:bool)
            n152 = Quotient & Remainder(x=w441, y=i64 2) -> (floor(x/y)=w437:i64)  [unwired: 1 out]
            n153 = In Range and Coerce(upper limit=w437, x=i64 5 ("upper limit"), lower limit=i64 1) -> (coerced(x)=w434:i64)  [unwired: 1 out]
            n154 = call <userlib>:"Get general message.vi"("timeout ms (1000)"=w434, "Mailbox ref in"=w435) -> ("error out"=w431:errorcluster, "Message"=w432:T12, "timed out?"=w430:bool)  [unwired: 4 in, 3 out]
            n155 = case shown="No Error" w431 {
              selector: w431 -> [_ w496]
              tunnel: [w452 TRUE] -> w424
              tunnel: [w451 w494] -> w428
              tunnel: w427 -> [w444 w493]
              tunnel: w432 -> [w450 _]
              tunnel: w430 -> [w447 _]
              tunnel: w429 -> [w445 _]
              tunnel: w433 -> [_ _]
              tunnel: [w443 w490] -> w426
              tunnel: [w442 APVSG_module_action."Exit"] -> w425
              frame No Error {
                # "Validation of command"
                # "Mailbox is OK"
                n156 = case shown="False" w447 {
                  tunnel: w450 -> [_ w468]
                  tunnel: [w455 w466] -> w449
                  tunnel: [THz_commands_enum."Ignore" ("Command") w464] -> w448
                  tunnel: ["Timed out" w465] -> w446
                  tunnel: w445 -> [_ w462]
                  frame True {
                    # "No message till time out"
                    n157 = xnode "Error Ring"() -> ("error out"=w455:errorcluster)
                  }
                  frame False {
                    w457 = T15[] [enum."Update", enum."Set parameters", enum."Disconnect"] items=["Ignore", "Connect", "Update", "Set parameters", "Disconnect", "End"] ("Command")
                    w458 = THz_commands_enum."Ignore" ("Command")
                    # "Message received in time\nValidation of command"
                    n158 = Unbundle By Name(w468) -> ("Topic"=w467:variant, "Content"=w465:variant)
                    n159 = Variant To Data(type=w458, Variant=w467) -> (data=w459:T15, error out=w466:errorcluster)  [unwired: 1 in]
                    n160 = Not Equal?(x=w459, y=w457) -> (x != y?=w461:bool[])
                    n161 = And Array Elements(Boolean array=w461) -> (logical AND=w460:bool)
                    n162 = Not Or(1:w460, 2:w462) -> (0:w463:bool)
                    n163 = Select(t=w458, s=w463, f=w459) -> (s? t:f=w464:T15)
                  }
                }
                n164 = case shown="No Error" w449 {
                  selector: w449 -> [_ w488]
                  tunnel: [_ FALSE] -> w452
                  tunnel: [w470 w487] -> w451
                  tunnel: w444 -> [w470 w484]
                  tunnel: w448 -> [w472 _]
                  tunnel: w446 -> [w469 _]
                  tunnel: [w469 w480] -> w443
                  tunnel: [w471 APVSG_module_action."Wait for event"] -> w442
                  frame No Error {
                    # "Correct command received"
                    n165 = case shown="\"Ignore\", Default" w472 {
                      tunnel: [APVSG_module_action."Wait for event" APVSG_module_action."Connect" APVSG_module_action."Query instr" APVSG_module_action."Set CW" APVSG_module_action."Disconnect" APVSG_module_action."Exit"] -> w471
                      frame "Ignore", Default {
                      }
                      frame "Connect" {
                      }
                      frame "Update" {
                      }
                      frame "Set parameters" {
                      }
                      frame "Disconnect" {
                      }
                      frame "End" {
                      }
                    }
                  }
                  frame Error {
                    # "Unknown command received"
                    n166 = Unbundle(w488) -> ("code"=w481:i32, "source"=w482:string)  [unwired: 1 out]
                    n167 = Unbundle By Name(w484) -> ("Logs"=w485:string[])
                    n168 = Format Into String(format string="Unknown command. Error: %d %s", w481, w482) -> (resulting string=w480:string)  [unwired: 2 in, 1 out]
                    n169 = call <userlib>:"Smart text logger.vi"("Message"=w480, "Logs in"=w485) -> ("Logs out"=w486:string[])  [unwired: 8 in, 1 out]
                    n170 = Bundle By Name(cluster=w484, "Logs"=w486) -> (w487:T2)
                  }
                }
              }
              frame Error {
                # "Queue Error"
                n171 = Unbundle(w496) -> ("code"=w498:i32, "source"=w497:string)  [unwired: 1 out]
                n172 = Format Into String(format string="Queue Error: %d %s" ("f"), w498, w497) -> (resulting string=w490:string)  [unwired: 2 in, 1 out]
                n173 = Unbundle By Name(w493) -> ("Logs"=w492:string[])
                n174 = call <userlib>:"Smart text logger.vi"("Message"=w490, "Logs in"=w492) -> ("Logs out"=w491:string[])  [unwired: 8 in, 1 out]
                n175 = Bundle By Name(cluster=w493, "Logs"=w491) -> (w494:T2)
              }
            }
          }
          frame True {
            n176 = Wait (ms)(milliseconds to wait=u32 1) -> ()  [unwired: 1 out]
          }
        }
      }
      frame "Wait for event" {
        n177 = Unbundle By Name(w510) -> ("Is standalone"=w518:bool, "Timer [ms]"=w515:i32, "Reset timer"=w516:bool)
        n178 = call <userlib>:"Periodic trigger ms.vi"("Reset (false)"=w516, "Period ms"=w515) -> ("Trigger"=w517:bool)  [unwired: 5 in]
        n179 = Bundle By Name(cluster=w510, "Reset timer"=FALSE) -> (w508:T2)
        n180 = And(x=w518, y=w517) -> (x .and. y?=w511:bool)
        n181 = Select(t=APVSG_module_action."Query instr", s=w511, f=APVSG_module_action."Check cmd") -> (s? t:f=w509:T9)
        n182 = case shown="\"Status\", Default" "APVSG tab" {
          tunnel: [w527 w546 w554 w563] -> w521
          tunnel: 0 -> [w526 w545 w553 w562]
          tunnel: w508 -> [w525 _ _ _]
          tunnel: [w524 _ _ _] -> w514
          tunnel: w509 -> [w523 w544 w552 w561]
          tunnel: [w522 w543 w551 w560] -> w506
          frame "Status", Default {
            n183 = event shown="[3] \"Enable ch 1\", \"Enable ch 2\": Value Change" {
              selector: _ -> [_ _ _ _]
              dyn-events: _ -> [_ _ _ _]
              timeout: w526 -> [_ _ _ _]
              tunnel: [w529 w534 APVSG_module_action."Exit" APVSG_module_action."Enable output"] -> w527
              tunnel: w525 -> [w530 _ _ _]
              tunnel: [w530 _ _ _] -> w524
              tunnel: w523 -> [w529 _ _ _]
              tunnel: [w528 w531 _ w539] -> w522
              tunnel: [w528 _ _ _] -> _
              event Timeout {
                n184 = event-data() -> ()  [unwired: 1 in, 3 out]
              }
              event "Connect btn": Value Change {
                n185 = event-data() -> ()  [unwired: 1 in, 6 out]
                n186 = Type Cast(x="VISA resource name") -> (*(type *) &x=w532:string)  [unwired: 1 in]
                n187 = Select(t=APVSG_module_action."Connect", s="Connect btn", f=APVSG_module_action."Disconnect") -> (s? t:f=w534:T9)
                n188 = To Variant(anything=w532) -> (Variant=w531:variant)
              }
              event "Exit APVSG btn": Value Change {
                n189 = event-data() -> ()  [unwired: 1 in, 6 out]
              }
              event "Enable ch 1", "Enable ch 2": Value Change {
                n190 = event-data() -> ()  [unwired: 1 in, 6 out]
                n191 = Build Array("Enable ch 1", "Enable ch 2") -> (w539:bool[])
              }
            }
          }
          frame "CW" {
            n192 = event shown="[1] \"CW settings\": Value Change" {
              selector: _ -> [_ _]
              dyn-events: _ -> [_ _]
              timeout: w545 -> [_ _]
              tunnel: [w547 APVSG_module_action."Set CW" ("f")] -> w546
              tunnel: w544 -> [w547 _]
              tunnel: [_ w548] -> w543
              event Timeout {
                n193 = event-data() -> ()  [unwired: 1 in, 3 out]
              }
              event "CW settings": Value Change {
                n194 = event-data() -> ()  [unwired: 1 in, 6 out]
                n195 = To Variant(anything="CW settings") -> (Variant=w548:variant)
              }
            }
          }
          frame "Sweep" {
            n196 = event shown="[1] \"Sweep table\": Value Change" {
              selector: _ -> [_ _]
              dyn-events: _ -> [_ _]
              timeout: w553 -> [_ _]
              tunnel: [w556 APVSG_module_action."Set sweep" ("f")] -> w554
              tunnel: w552 -> [w556 _]
              tunnel: [variant w557] -> w551
              event Timeout {
                n197 = event-data() -> ()  [unwired: 1 in, 3 out]
              }
              event "Sweep table": Value Change {
                n198 = event-data() -> ()  [unwired: 1 in, 6 out]
                n199 = To Variant(anything="Sweep table") -> (Variant=w557:variant)
              }
            }
          }
          frame "Arbitrary" {
            n200 = event shown="[1] \"Waveform files\": Value Change" {
              selector: _ -> [_ _]
              dyn-events: _ -> [_ _]
              timeout: w562 -> [_ _]
              tunnel: [w564 _] -> w563
              tunnel: w561 -> [w564 _]
              tunnel: [_ w565] -> w560
              event Timeout {
                n201 = event-data() -> ()  [unwired: 1 in, 3 out]
              }
              event "Waveform files": Value Change {
                n202 = event-data() -> ()  [unwired: 1 in, 6 out]
                n203 = To Variant(anything="Waveform files") -> (Variant=w565:variant)
              }
            }
          }
        }
      }
      frame "Connect" {
        # "Connect to instrument. Report to supermodule if possible."
        n204 = Variant To Data(type="", Variant=w593) -> (data=w570:string)  [unwired: 1 in, 1 out]
        n205 = Bundle By Name(cluster=w573, "Connection"=w570) -> (w572:T1)
        n206 = call "Initialize APSVG.vi"("MW generator constants"=w572) -> ("error out"=w568:errorcluster, "MW generator constants out"=w582:T1)  [unwired: 5 in, 4 out]
        n207 = Unbundle By Name(w586) -> ("Logs"=w583:string[], "Supramodule"=w590:T3, "Module name"=w591:string, "Is standalone"=w592:bool)
        n208 = Unbundle By Name(w582) -> ("Device name"=w578:string, "Description"=w577:string, "Connection"=w576:string, "Connected"=w567:bool)
        "Is connected" <- w567
        n209 = call <vilib>:"Space Constant.vi"() -> ("String"=w575:string)
        n210 = Concatenate Strings(w578, w575, w577, "connected by " ("String"), w576) -> (w581:string)
        n211 = Select(t=w581, s=w567, f="Not connected") -> (s? t:f=w579:string)
        n212 = property on="VISA resource name" class="VISAName"(error in=w568, "DisabledEnum"=T16."Disabled and Grayed Out" ("Disabled")) -> ()  [unwired: 1 in, 2 out]
        n213 = case shown="False" w592 {
          tunnel: w591 -> [w597 _]
          tunnel: w589 -> [w596 _]
          tunnel: w582 -> [w595 _]
          tunnel: w590 -> [w594 _]
          frame False {
            # "Report last action"
            n214 = call <userlib>:"Send general mesage.vi"("Content"=w595, "Topic"=w596, "Sender"=w597, "Mailbox ref in"=w594) -> ()  [unwired: 5 in, 3 out]
          }
          frame True {
            # "No module to report"
          }
        }
        n215 = local write "Connect btn"(w567) -> ()
        n216 = call <userlib>:"Smart text logger.vi"("Message"=w579, "Logs in"=w583) -> ("Logs out"=w584:string[])  [unwired: 8 in, 1 out]
        n217 = Bundle By Name(cluster=w586, "Logs"=w584) -> (w585:T2)
      }
      frame "Disconnect" {
        # "Disconnect from the instrument. Report to supermodule if possible."
        n218 = Unbundle By Name(w604) -> ("Device name"=w605:string, "Connection"=w607:string, "Connected"=w606:bool)
        n219 = case shown="True" w606 {
          selector: w606 -> [w619 w622]
          tunnel: w607 -> [_ w624]
          tunnel: [w619 w621] -> w599
          tunnel: ["already disconnected" "disconnected"] -> w602
          tunnel: [_ w620] -> w600
          frame False {
          }
          frame True {
            n220 = VISA Close(VISA resource name=w624) -> (error out=w620:errorcluster)  [unwired: 1 in]
            n221 = Not(x=w622) -> (.not. x?=w621:bool)
          }
        }
        n222 = Unbundle By Name(w611) -> ("Logs"=w608:string[], "Supramodule"=w615:T3, "Module name"=w616:string, "Is standalone"=w617:bool)
        n223 = Concatenate Strings(w605, w602) -> (w598:string)
        n224 = property on="VISA resource name" class="VISAName"(error in=w600, "DisabledEnum"=T16."Enabled" ("Disabled")) -> ()  [unwired: 1 in, 2 out]
        n225 = case shown="False" w617 {
          tunnel: w616 -> [w628 _]
          tunnel: w614 -> [w627 _]
          tunnel: w615 -> [w626 _]
          tunnel: w598 -> [w625 _]
          frame False {
            # "Report last action"
            n226 = call <userlib>:"Send general mesage.vi"("Content"=w625, "Topic"=w627, "Sender"=w628, "Mailbox ref in"=w626) -> ()  [unwired: 5 in, 3 out]
          }
          frame True {
            # "No module to report"
          }
        }
        n227 = Bundle By Name(cluster=w604, "Connected"=w599) -> (w603:T1)
        n228 = local write "Connect btn"(w599) -> ()
        n229 = call <userlib>:"Smart text logger.vi"("Message"=w598, "Logs in"=w608) -> ("Logs out"=w609:string[])  [unwired: 8 in, 1 out]
        n230 = Bundle By Name(cluster=w611, "Logs"=w609) -> (w610:T2)
      }
      frame "Query instr" {
        # "This case is for periodic quering of instrument state, properties, settings. It is initiated by command or timeout event."
        n231 = Unbundle By Name(w636) -> ("Connection"=w644:string)
        n232 = Concatenate Strings("OUTP:STAT?" ("write buffer"), "\n") -> (w638:string)
        n233 = VISA Write(VISA resource name=w644, write buffer=w638) -> (VISA resource name out=w642:refnum<visa-resource-name>, error out=w645:errorcluster)  [unwired: 1 in, 1 out]
        n234 = VISA Read(VISA resource name=w642, byte count=u32 1024, error in (no error)=w645) -> (read buffer=w637:string, error out=w630:errorcluster)  [unwired: 2 out]
        n235 = call <vilib>:"Trim Whitespace.vi"("string"=w637) -> ("trimmed string"=w641:string)  [unwired: 1 in]
        n236 = Not(x=w630) -> (.not. x?=w629:bool)
        n237 = case shown="\"1\"" w641 {
          tunnel: [FALSE FALSE TRUE] -> _
          frame "False", Default {
          }
          frame "0" {
          }
          frame "1" {
          }
        }
        n238 = Unbundle By Name(w635) -> ("Supramodule"=w634:T3, "Module name"=w633:string)
        n239 = Bundle By Name(cluster=w636, "Connected"=w629) -> (w631:T1)  [unwired: 2 in]
        n240 = call <userlib>:"Send general mesage.vi"("Content"=w631, "Topic"=w632, "Sender"=w633, "Mailbox ref in"=w634) -> ()  [unwired: 5 in, 3 out]
        n241 = Bundle By Name(cluster=w635, "Reset timer"=TRUE) -> (w646:T2)
      }
      frame "Set CW" {
        n242 = Unbundle By Name(w668) -> ("Module name"=w651:string, "Is standalone"=w656:bool, "Supramodule"=w655:T3, "Logs"=w661:string[])
        n243 = Variant To Data(type=T4 [] ("CW settings 2"), Variant=w671) -> (data=w669:T4, error out=w662:errorcluster)  [unwired: 1 in]
        n244 = Unbundle By Name(w667) -> ("Connection"=w663:string)  [unwired: 1 out]
        n245 = for {
          tunnel: w669 -> [w694] mode=indexing
          tunnel: [w699] -> _
          tunnel: w663 -> [w691]
          shift-right: [w700] -> w660
          shift-left: w662 -> [w690]
          i -> [w693]
          n246 = Unbundle(w694) -> ("Frequency (GHz)"=w695:dbl, "Amplitude (dBm)"=w696:dbl)
          n247 = Increment(x=w693) -> (x+1=w692:i32)
          n248 = To Unsigned Word Integer(number=w692) -> (unsigned 16bit integer=w689:u16)
          n249 = call <instrlib>:"Select default channel.vi"("error in (no error)"=w690, "Channel (1)"=w689, "VISA resource name"=w691) -> ("error out"=w697:errorcluster, "VISA resource out"=w698:refnum<visa-resource-name>)  [unwired: 7 in]
          n250 = call <instrlib>:"Configure RF Output.vi"("VISA resource name"=w698, "Frequency (100)"=w695, "error in (no error)"=w697, "Power Level (0.00 dBm)"=w696) -> ("VISA resource name out"=w699:refnum<visa-resource-name>, "error out"=w700:errorcluster)  [unwired: 10 in]
        }
        n251 = case shown="No Error" w660 {
          selector: w660 -> [_ w685]
          tunnel: w661 -> [w679 w684]
          tunnel: [w680 w683] -> w659
          tunnel: [w677 w682] -> w652
          tunnel: [w678 w681] -> w657
          frame No Error {
            w677 = "APVSG set to CW mode" ("Message")
            n252 = call <userlib>:"Smart text logger.vi"("Message"=w677, "Logs in"=w679) -> ("Repeats twice?"=w678:bool, "Logs out"=w680:string[])  [unwired: 8 in]
          }
          frame Error {
            n253 = Unbundle(w685) -> ("code"=w688:i32, "source"=w687:string)  [unwired: 1 out]
            n254 = Format Into String(format string="Queue Error: %d %s" ("f"), w688, w687) -> (resulting string=w682:string)  [unwired: 2 in, 1 out]
            n255 = call <userlib>:"Smart text logger.vi"("Message"=w682, "Logs in"=w684) -> ("Repeats twice?"=w681:bool, "Logs out"=w683:string[])  [unwired: 8 in]
          }
        }
        n256 = Or(x=w656, y=w657) -> (x .or. y?=w654:bool)
        n257 = case shown="False" w654 {
          tunnel: w655 -> [w673 _]
          tunnel: w653 -> [w676 _]
          tunnel: w652 -> [w675 _]
          tunnel: w651 -> [w674 _]
          frame False {
            n258 = call <userlib>:"Send general mesage.vi"("Content"=w675, "Topic"=w676, "Sender"=w674, "Mailbox ref in"=w673) -> ()  [unwired: 5 in, 3 out]
          }
          frame True {
          }
        }
        n259 = Bundle By Name(cluster=w667, "Operation mode"=enum16{"Disabled", "CW", "Arbitrary", "Sweep"}."CW", "Last settings"=w652) -> (w665:T1)
        n260 = Bundle By Name(cluster=w668, "Logs"=w659) -> (w666:T2)
      }
      frame "Set sweep" {
      }
      frame "Set waveform" {
      }
      frame "Enable output" {
        n261 = Unbundle By Name(w711) -> ("Connection"=w705:string, "Connected"=w710:bool)
        n262 = Unbundle By Name(w707) -> ()  [unwired: 3 out]
        n263 = case shown="True" w710 {
          tunnel: w712 -> [_ w717]
          tunnel: w705 -> [_ w713]
          frame False {
          }
          frame True {
            n264 = Variant To Data(type=bool[] [], Variant=w717) -> (data=w715:bool[], error out=w714:errorcluster)  [unwired: 1 in]
            n265 = for {
              tunnel: w715 -> [w723] mode=indexing
              shift-right: [w719] -> _
              shift-left: w714 -> [w722]
              tunnel: w713 -> [w718]
              i -> [w721]
              stop <- w719 stop-if-true
              n266 = Increment(x=w721) -> (x+1=w720:i32)
              n267 = call <instrlib>:"Select default channel.vi"("error in (no error)"=w722, "Channel (1)"=w720, "VISA resource name"=w718) -> ("error out"=w724:errorcluster, "VISA resource out"=w725:refnum<visa-resource-name>)  [unwired: 7 in]
              n268 = call <instrlib>:"Enable Output.vi"("Enable Output (T: Enable)"=w723, "error in (no error)"=w724, "VISA resource name"=w725) -> ("error out"=w719:errorcluster)  [unwired: 7 in, 1 out]
            }
            n269 = case shown="True" {
              selector: _ -> [_ _]
              frame False {
              }
              frame True {
              }
            }
          }
        }
        n270 = Get Date/Time In Seconds() -> (seconds since 1Jan1904=w706:timestamp)
        n271 = Bundle By Name(cluster=w711) -> (w709:T1)  [unwired: 3 in]
        n272 = Bundle By Name(cluster=w707, "Last change"=w706) -> (w708:T2)  [unwired: 1 in]
      }
    }
    "Modul status" <- w382
    "Instrument status" <- w377
  }
  n273 = flat-sequence {
    tunnel: w6 -> [w729]
    tunnel: [w728] -> _
    frame #0 {
      n274 = Bundle By Name(cluster=w729, "Stopped?"=TRUE) -> (w728:T7)
      n275 = Wait (ms)(milliseconds to wait=u32 100) -> ()  [unwired: 1 out]
    }
  }
